vi "Report Project.vi"(7 "Memory":T1, 8 "error in (no error)":errorcluster {"code" format="Error %.0f"}, 9 "Msg Chain":string, 10 "Project Doc":refnum<class "Project Documentation.lvclass">, 11 "VIDoc Printer In":refnum<class "VIDoc Printer.lvclass">) -> (0 "error out":errorcluster {"code" format="Error %.0f"}, 3 "VIDoc Printer Out":refnum<class "VIDoc Printer.lvclass">)   [LabVIEW 2023, in "VIDoc Printer.lvlib" / "VIDoc Printer.lvclass"]
uses:
  VIDoc Printer.lvclass
  Parsing/Project Documentation/Project Documentation.lvclass
  Parsing/TypeDefs/Memory Size Cluster.ctl
  VIDoc Printer.lvclass/VIDoc Printer.ctl
  Parsing/Project Documentation/Project Documentation.lvclass/Project Documentation.ctl
  Parsing/Project Documentation/Get Name.vi
  Accessors/Get Projects Enabled.vi
  Accessors/Process Actions/Get Process Project Actions.vi
  Parsing/VIDoc Parsing.lvlib
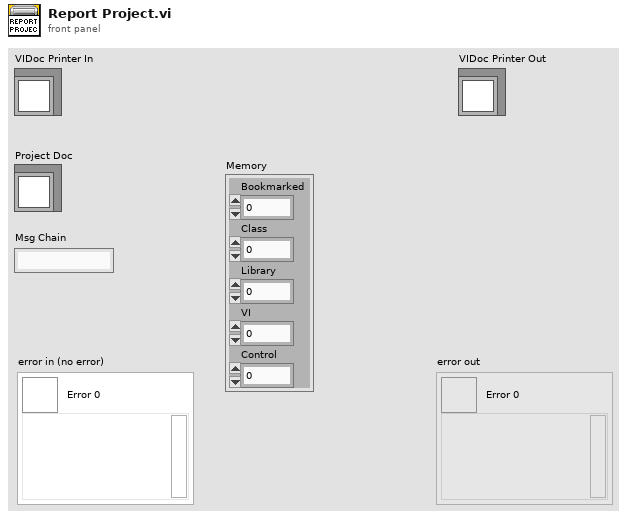
[diagram p1: front panel]
types:
  T1 = typedef "VIDoc Parsing.lvlib/Memory Size Cluster.ctl" = cluster{"Bookmarked":dbl, "Class":dbl, "Library":dbl, "VI":dbl, "Control":dbl}
  T2 = typedef "VIDoc Printer.lvlib/VIDoc Printer.lvclass/Process Project Enum.ctl" = enum16{"Name", "Description", "Memory", "Options", "Symbols"}
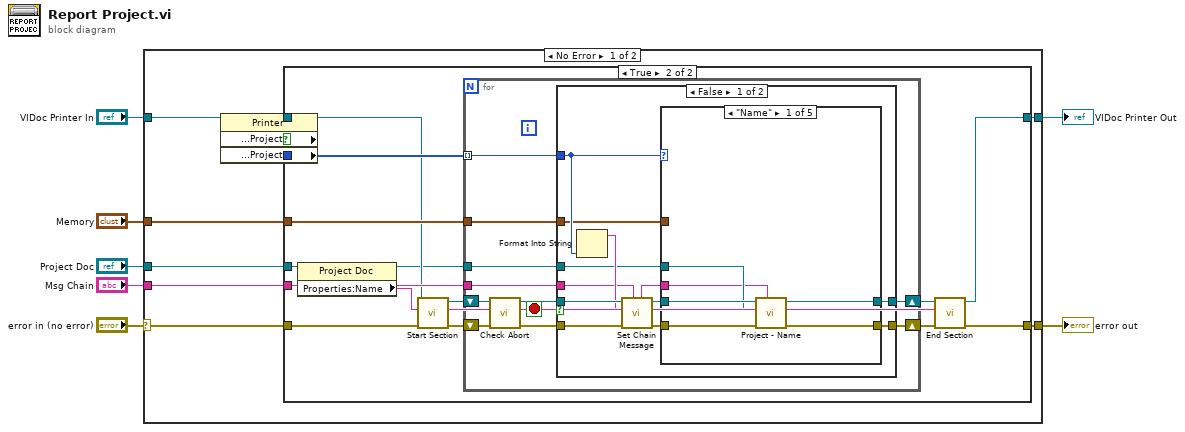
[diagram p0: block diagram]
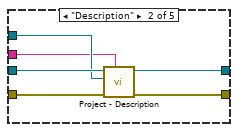
[diagram p3: hidden frame]
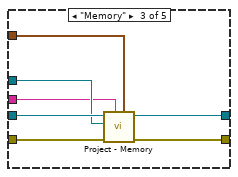
[diagram p4: hidden frame]
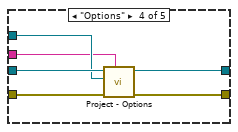
[diagram p5: hidden frame]
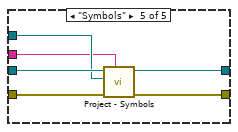
[diagram p6: hidden frame]
diagram:
  n1 = case shown="No Error" "error in (no error)" {
    selector: "error in (no error)" -> [w17 w91]
    tunnel: [w14 w91] -> w6
    tunnel: [w11 w90] -> w4
    tunnel: "VIDoc Printer In" -> [w15 w90]
    tunnel: "Msg Chain" -> [w16 _]
    tunnel: "Project Doc" -> [w13 _]
    tunnel: "Memory" -> [w10 _]
    frame No Error {
      n2 = property class="Printer"(reference=w15) -> (reference out=w12:refnum<class "VIDoc Printer.lvclass">, "Properties:Settings:Enabled Sections:Projects"=w9:bool, "Properties:Process Lists:Projects"=w8:T2[])  [unwired: 1 in, 1 out]
      n3 = case shown="True" w9 {
        tunnel: w17 -> [w19 w27]
        tunnel: w16 -> [_ w33]
        tunnel: [w19 w21] -> w14
        tunnel: w13 -> [_ w32]
        tunnel: w12 -> [w18 w29]
        tunnel: [w18 w23] -> w11
        tunnel: w10 -> [_ w31]
        tunnel: w8 -> [_ w30]
        frame False {
        }
        frame True {
          n4 = property class="Project Doc"(reference=w32) -> (reference out=w25:refnum<class "Project Documentation.lvclass">, "Properties:Name"=w20:string)  [unwired: 1 in, 1 out]
          n5 = call-dynamic "Start Section.vi"("error in (no error)"=w27, "Section"=w20, "VIDoc Printer In"=w29) -> ("error out"=w26:errorcluster, "VIDoc Printer Out"=w28:refnum<class "VIDoc Printer.lvclass">)  [unwired: 7 in]
          n6 = for {
            shift-right: [w42] -> w22
            shift-left: w26 -> [w44]
            tunnel: w33 -> [w38]
            tunnel: w25 -> [w37]
            tunnel: w31 -> [w36]
            shift-right: [w40] -> w24
            shift-left: w28 -> [w43]
            tunnel: w30 -> [w35] mode=indexing
            stop <- w34 stop-if-true
            n7 = call "Check Abort.vi"("error in (no error)"=w44, "VIDoc Printer In"=w43) -> ("error out"=w41:errorcluster, "Abort?"=w34:bool, "VIDoc Printer Out"=w39:refnum<class "VIDoc Printer.lvclass">)  [unwired: 7 in]
            n8 = case shown="False" w34 {
              tunnel: [w56 w89] -> w42
              tunnel: w41 -> [w53 w89]
              tunnel: [w55 w88] -> w40
              tunnel: w39 -> [w51 w88]
              tunnel: w38 -> [w45 _]
              tunnel: w37 -> [w48 _]
              tunnel: w36 -> [w47 _]
              tunnel: w35 -> [w50 _]
              frame False {
                n9 = Format Into String(w50) -> (resulting string=w49:string)  [unwired: 3 in, 1 out]
                n10 = call "Set Chain Message.vi"("Msg Chain"=w45, "error in (no error)"=w53, "New"=w49, "VIDoc Printer In"=w51) -> ("error out"=w54:errorcluster, "VIDoc Printer Out"=w52:refnum<class "VIDoc Printer.lvclass">, "Msg Chain out"=w46:string)  [unwired: 5 in]
                n11 = case shown="\"Name\"" w50 {
                  tunnel: w54 -> [w61 w67 w74 w80 w86]
                  tunnel: [w59 w65 w72 w78 w84] -> w56
                  tunnel: w52 -> [w62 w68 w75 w81 w87]
                  tunnel: [w60 w66 w73 w79 w85] -> w55
                  tunnel: w48 -> [w58 w64 w71 w77 w83]
                  tunnel: w47 -> [_ _ w70 _ _]
                  tunnel: w46 -> [w57 w63 w69 w76 w82]
                  frame "Name" {
                    n12 = call-dynamic "Project - Name.vi"("Msg Chain"=w57, "error in (no error)"=w61, "Project Doc"=w58, "VIDoc Printer In"=w62) -> ("error out"=w59:errorcluster, "VIDoc Printer Out"=w60:refnum<class "VIDoc Printer.lvclass">)  [unwired: 6 in]
                  }
                  frame "Description" {
                    n13 = call-dynamic "Project - Description.vi"("Msg Chain"=w63, "error in (no error)"=w67, "Project Doc"=w64, "VIDoc Printer In"=w68) -> ("error out"=w65:errorcluster, "VIDoc Printer Out"=w66:refnum<class "VIDoc Printer.lvclass">)  [unwired: 6 in]
                  }
                  frame "Memory" {
                    n14 = call-dynamic "Project - Memory.vi"("Memory"=w70, "Msg Chain"=w69, "error in (no error)"=w74, "Project Doc"=w71, "VIDoc Printer In"=w75) -> ("error out"=w72:errorcluster, "VIDoc Printer Out"=w73:refnum<class "VIDoc Printer.lvclass">)  [unwired: 5 in]
                  }
                  frame "Options" {
                    n15 = call-dynamic "Project - Options.vi"("Msg Chain"=w76, "error in (no error)"=w80, "Project Doc"=w77, "VIDoc Printer In"=w81) -> ("error out"=w78:errorcluster, "VIDoc Printer Out"=w79:refnum<class "VIDoc Printer.lvclass">)  [unwired: 6 in]
                  }
                  frame "Symbols" {
                    n16 = call-dynamic "Project - Symbols.vi"("Msg Chain"=w82, "error in (no error)"=w86, "Project Doc"=w83, "VIDoc Printer In"=w87) -> ("error out"=w84:errorcluster, "VIDoc Printer Out"=w85:refnum<class "VIDoc Printer.lvclass">)  [unwired: 6 in]
                  }
                }
              }
              frame True {
              }
            }
          }
          n17 = call-dynamic "End Section.vi"("error in (no error)"=w22, "Section"=w20, "VIDoc Printer In"=w24) -> ("error out"=w21:errorcluster, "VIDoc Printer Out"=w23:refnum<class "VIDoc Printer.lvclass">)  [unwired: 7 in]
        }
      }
    }
    frame Error {
    }
  }
  "error out" <- w6
  "VIDoc Printer Out" <- w4
